vi "SR430.get scan status.vi"(0 "i ref in":refnum<vi>, 5 "error in (no error)":errorcluster) -> (14 "i ref out":refnum<vi>, 16 "scanStatus":bool, 19 "error out":errorcluster)   [LabVIEW 2014, in "SR430.lvlib"]
doc: "determines, if the number of records accumulated equals the number of records per scan (set-value)."
uses:
  SR430.lvlib
  CSCore/CSApplicationBaseClasses/MCSBase/MCSBase.directionType.ctl
  CSCore/CSApplicationBaseClasses/MCSBase/MCSBase.serviceType.ctl
  CSlibraries/UtilityLib/UtilityLib.valueStatus.ctl
  CSCore/CSSystem/CoreDefs/CoreDefs.error_type.ctl
  CSinstr.lib/Sr430/SR430Driver.lvlib
  CSCore/CSSystem/CoreLib/CoreLib.lvlib
  CSCore/CSApplicationBaseClasses/MCSBase/MCSBase.lvlib
  CSlibraries/UtilityLib/UtilityLib.lvlib
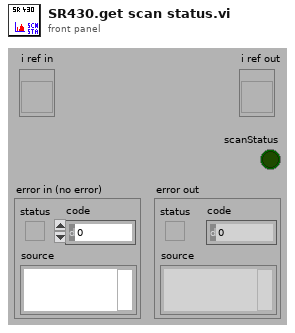
[diagram p1: front panel]
types:
  T1 = typedef "UtilityLib.lvlib/UtilityLib.valueStatus.ctl" = enum16{"no info available", "stand by/off", "on", "warning", "alarm/malfunction", "not implemented", "user action required", "important information", "system default", "control default", "indicator default", "button default"}
  T2 = typedef "MCSBase.lvlib/MCSBase.serviceType.ctl" = enum16{"counts", "totalCounts", "binWidth", "nOfBins", "nOfRecords", "status", "discrLevel", "discrSlope", "triggerLevel", "triggerSlope"}
  T3 = typedef "MCSBase.lvlib/MCSBase.directionType.ctl" = enum16{"unknown", "update actual value", "update nominal value", "update both"}
  T4 = typedef "CoreDefs.error_type.ctl" = enum16{"no error", "can't load process", "can't unload process", "process does not exist", "can't install process", "can't remove process", "unknown function", "time out", "can't execute function", "duplicate queue name", "super not found", "caller queue invalid", "can't ping process", "unknown error", "VISA Error", "VISA timeout", "GPIB timeout", "GPIB error", "communication error", "data type mismatch", "can't read data from OPC server", "can't write data to OPC server", "OET error", "function not implemented", "process already exists", "invalid Shared Variable name", "error writing Shared Variable", "error reading Shared Variable", "invalid client name", "corrupt database", "unknown class", "call not authorized", "parameter out of range", "OET timeout: can't get data to modify", "invalid queue name", "requested operation incompatible with current state", "event undefined", "event disabled", "state undefined", "caller is not a friend", "EventBuilder: bad eventID", "EventBuilder: no DAQ devices", "a thread must not stop itself", "UNUSED ELEMENT4", "DiscArchiver: eventData incomplete", "DiscArchiver: eventData does not belong to run", "DiscArchiver: can't open file", "DiscArchiver: can't write to file", "DiscArchiver: available disc space low", "can't acquire semaphore", "error reading data from database", "notifier object is not existing", "can't register process", "can't unregister process", "illegal event type", "object disabled", "object already exists", "can't change state", "Instrument not found", "no connection to remote node", "invalid reference", "N/A", "UNUSED ELEMENT 1", "element not found", "illegal TCP/IP connection detected", "object does not exist", "invalid access ID", "unknown CS system", "invalid privilige", "unsupported data type", "unsupported server type", "IO server already exists", "Shared Variable already exists"}
  T5 = typedef "SR430Driver.lvlib/SR430_VISA Control.ctl" = cluster{"VISA resource name":refnum<visa-resource-name>}
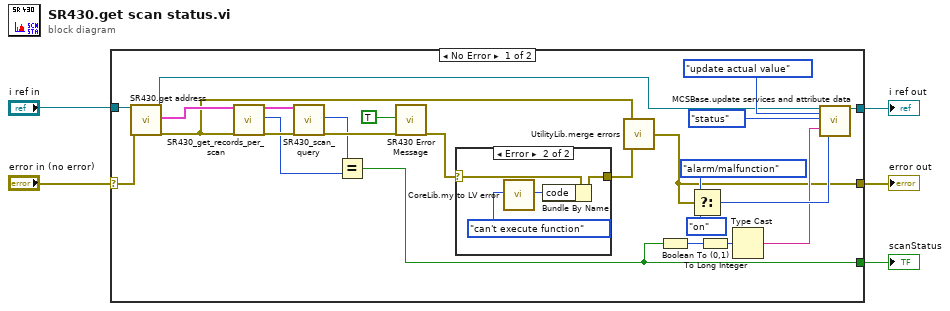
[diagram p0: block diagram]
diagram:
  n1 = case shown="No Error" "error in (no error)" {
    selector: "error in (no error)" -> [w18 w35]
    tunnel: "i ref in" -> [w29 w36]
    tunnel: [w8 w35] -> w4
    tunnel: [w9 w36] -> w3
    tunnel: [w7 _] -> w2
    frame No Error {
      n2 = call "SR430.get address.vi"("i ref in"=w29, "error in (no error)"=w18) -> ("i ref out"=w6:refnum<vi>, "address"=w28:T5, "error out"=w27:errorcluster)  [unwired: 15 in]
      n3 = call "SR430_get_records_per_scan.vi"("address"=w28, "error in (no error)"=w27) -> ("addressOut"=w25:T5, "recordsPerScan"=w21:i32, "error out"=w24:errorcluster)  [unwired: 15 in]
      n4 = call "SR430_scan_query.vi"("address"=w25, "error in (no error)"=w24) -> ("recordsAccumulated"=w22:i32, "error out"=w23:errorcluster)  [unwired: 15 in, 1 out]
      n5 = Equal?(x=w22, y=w21) -> (x = y?=w7:bool)
      n6 = call "SR430 Error Message.vi"("addMessageToSource"=TRUE ("add message to source"), "error in (no error)"=w23) -> ("error out"=w26:errorcluster)  [unwired: 14 in, 3 out]
      n7 = case shown="Error" w26 {
        selector: w26 -> [w30 w34]
        tunnel: [w30 w31] -> w19
        frame No Error {
        }
        frame Error {
          n8 = call "CoreLib.my to LV error.vi"("ErrorTypes"=CoreDefs.error_type."can't execute function") -> ("LV error code"=w33:i32)  [unwired: 17 in, 1 out]
          n9 = Bundle By Name(cluster=w34, "code"=w33) -> (w31:errorcluster)
        }
      }
      n10 = call "UtilityLib.merge errors.vi"("error2 (no error)"=w19, "error1 (no error)"=w27) -> ("error out"=w8:errorcluster)
      n11 = Boolean To (0,1)(Boolean=w7) -> (0, 1=w17:i16)
      n12 = Select(t=UtilityLib.valueStatus."alarm/malfunction" ("quality"), s=w8, f=UtilityLib.valueStatus."on") -> (s? t:f=w12:T1)
      n13 = To Long Integer(number=w17) -> (32bit integer=w10:i32)
      n14 = Type Cast(x=w10) -> (*(type *) &x=w11:string)  [unwired: 1 in]
      n15 = call "MCSBase.update services and attribute data.vi"("i ref in"=w6, "direction"=MCSBase.directionType."update actual value", "service"=MCSBase.serviceType."status", "value"=w11, "quality"=w12) -> ("i ref out"=w9:refnum<vi>)  [unwired: 12 in, 2 out]
    }
    frame Error {
    }
  }
  "error out" <- w4
  "i ref out" <- w3
  "scanStatus" <- w2
